vi "Add Config File Dependency.vi"(8 "error in (no error)":errorcluster, 11 "Item Ref in":T1 format="%.0x") -> (0 "error out":errorcluster, 2 "configuration file set?":bool, 3 "Device Ref out":T1 format="%.0x")   [LabVIEW 2021, in "DSF System Explorer.lvlib"]
uses:
  DSF System Explorer.lvlib
  <vilib>/NI VeriStand/Custom Device API/Custom Device Item Ref.ctl
  <vilib>/NI VeriStand/Custom Device API/Custom Device File Dependency.ctl
  <vilib>/NI VeriStand/Custom Device API/Path Specification.ctl
  <vilib>/NI VeriStand/Custom Device API/Path Type.ctl
  <vilib>/NI VeriStand/Custom Device API/Custom Device Supported Target.ctl
  <vilib>/NI VeriStand/Custom Device API/Get Item Property (Path).vi
  <vilib>/NI VeriStand/Custom Device API/Custom Device API.lvlib
  Shared/DSF Shared.lvlib
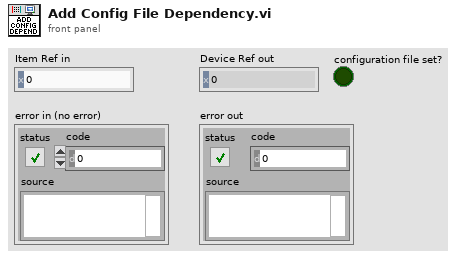
[diagram p1: front panel]
types:
  T1 = typedef "Custom Device API.lvlib/Custom Device Item Ref.ctl" = u64
  T2 = typedef "Custom Device API.lvlib/Custom Device Supported Target.ctl" = enum16{"All", "PharLap", "VxWorks", "Windows", "Linux_32_ARM", "Linux_x64", "PharLap & Windows", "PharLap & VxWorks", "VxWorks & Windows"}
  T3 = typedef "Custom Device API.lvlib/Path Type.ctl" = enum16{"Absolute", "To Base", "To Common Data Dir", "To Application Data Dir"}
  T4 = typedef "Custom Device API.lvlib/Custom Device File Dependency.ctl" = cluster{"Source":T5, "RT Destination":path, "ForceDownload?":bool, "SupportedTarget":T2, "Version":string}
  T5 = typedef "Custom Device API.lvlib/Path Specification.ctl" = cluster{"Path":path, "Type":T3}
  T6 = typedef "Custom Device API.lvlib/Custom Device Target Type.ctl" = enum16{"PharLap", "VxWorks", "Windows", "Linux_32_ARM", "Linux_x64"}
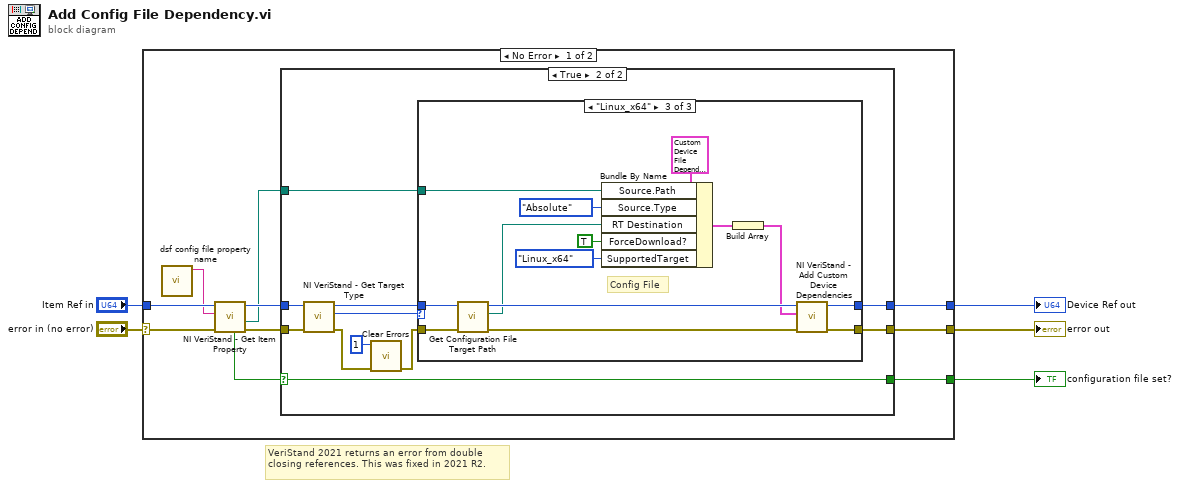
[diagram p0: block diagram]
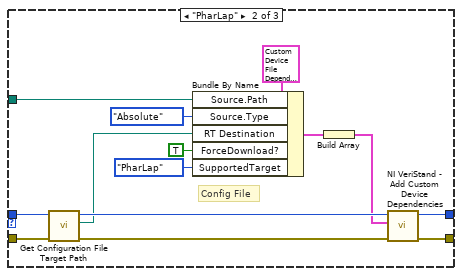
[diagram p4: hidden frame]
diagram:
  # "VeriStand 2021 returns an error from double closing references. This was fixed in 2021 R2."
  n1 = case shown="No Error" "error in (no error)" {
    selector: "error in (no error)" -> [w12 w61]
    tunnel: [w15 w60] -> w5
    tunnel: [w14 w61] -> w4
    tunnel: "Item Ref in" -> [w13 w60]
    tunnel: [w6 _] -> w1
    frame No Error {
      n2 = call "dsf config file property name.vi"() -> ("file path property name"=w9:string)  [unwired: 11 in]
      n3 = call-poly <vilib>:"NI VeriStand - Get Item Property.vi"("error in (no error)"=w12, "Property Name"=w9, "Item Ref in"=w13) -> ("error out"=w10:errorcluster, "Value"=w8:path, "Item Ref out"=w11:T1, "Found?"=w7:bool)  [unwired: 5 in]
      n4 = case shown="True" w7 {
        selector: w7 -> [w16 w22]
        tunnel: [w18 w27] -> w15
        tunnel: [w17 w26] -> w14
        tunnel: w11 -> [w18 w25]
        tunnel: w10 -> [w17 w24]
        tunnel: w8 -> [_ w23]
        tunnel: [w16 w22] -> w6
        frame False {
        }
        frame True {
          n5 = call <vilib>:"NI VeriStand - Get Target Type.vi"("error in (no error)"=w24, "Item Ref in"=w25) -> ("error out"=w20:errorcluster, "Target Type"=w29:T6, "Item Ref out"=w28:T1)  [unwired: 7 in]
          n6 = call <vilib>:"Clear Errors.vi"("error in (no error)"=w20, "specific error code to clear (0: all)"=1) -> ("error out"=w19:errorcluster)  [unwired: 4 in, 1 out]
          n7 = case shown="\"Linux_x64\"" w29 {
            tunnel: [w31 w43 w57] -> w26
            tunnel: [w30 w42 w56] -> w27
            tunnel: w28 -> [w30 w45 w59]
            tunnel: w19 -> [w31 w44 w58]
            tunnel: w23 -> [_ w41 w55]
            frame "Windows", Default {
              # "Don't add dependency for Windows or unsupported target type."
            }
            frame "PharLap" {
              # "Config File"
              n8 = call "Get Configuration File Target Path.vi"("error in (no error)"=w44, "Item Ref in"=w45) -> ("error out"=w35:errorcluster, "configuration target path"=w33:path, "Item Ref out"=w34:T1)  [unwired: 7 in]
              n9 = Bundle By Name(cluster=T4 {"Source"={"Path"=path "", "Type"=enum."Absolute"}, "RT Destination"=path "", "ForceDownload?"=FALSE, "SupportedTarget"=enum."PharLap", "Version"=""} ("Dependencies"), "Source.Path"=w41, "Source.Type"=Path_Type."Absolute", "RT Destination"=w33, "ForceDownload?"=TRUE, "SupportedTarget"=Custom_Device_Supported_Target."PharLap") -> (w36:T4)
              n10 = Build Array(w36) -> (w32:T4[])
              n11 = call <vilib>:"NI VeriStand - Add Custom Device Dependencies.vi"("error in (no error)"=w35, "Dependencies"=w32, "Device Ref in"=w34) -> ("error out"=w43:errorcluster, "Device Ref out"=w42:T1)  [unwired: 7 in]
            }
            frame "Linux_x64" {
              # "Config File"
              n12 = call "Get Configuration File Target Path.vi"("error in (no error)"=w58, "Item Ref in"=w59) -> ("error out"=w49:errorcluster, "configuration target path"=w47:path, "Item Ref out"=w48:T1)  [unwired: 7 in]
              n13 = Bundle By Name(cluster=T4 {"Source"={"Path"=path "", "Type"=enum."Absolute"}, "RT Destination"=path "", "ForceDownload?"=FALSE, "SupportedTarget"=enum."PharLap", "Version"=""} ("Dependencies"), "Source.Path"=w55, "Source.Type"=Path_Type."Absolute", "RT Destination"=w47, "ForceDownload?"=TRUE, "SupportedTarget"=Custom_Device_Supported_Target."Linux_x64") -> (w50:T4)
              n14 = Build Array(w50) -> (w46:T4[])
              n15 = call <vilib>:"NI VeriStand - Add Custom Device Dependencies.vi"("error in (no error)"=w49, "Dependencies"=w46, "Device Ref in"=w48) -> ("error out"=w57:errorcluster, "Device Ref out"=w56:T1)  [unwired: 7 in]
            }
          }
        }
      }
    }
    frame Error {
    }
  }
  "Device Ref out" <- w5
  "error out" <- w4
  "configuration file set?" <- w1
